vi "readUDP.vi"(8 "error in (no error)":errorcluster, 11 "Mockbus in":refnum<class "Mockbus.lvclass">) -> (0 "error out":errorcluster, 1 "CommandAvailable":bool, 2 "UDP Command":T1, 3 "Mockbus out":refnum<class "Mockbus.lvclass">)   [LabVIEW 2015, in "Mockbus.lvclass"]
uses:
  Mockbus.lvclass
  Typedefs/UDPCommand.ctl
  Mockbus.lvclass/Mockbus.ctl
  Typedefs/RTTypeDefs.lvlib
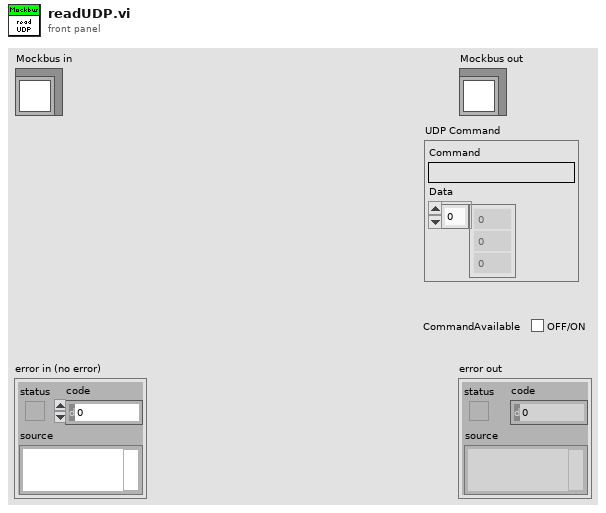
[diagram p1: front panel]
types:
  T1 = typedef "RTTypeDefs.lvlib/UDPCommand.ctl" = cluster{"Command":string, "Data":u8[]}
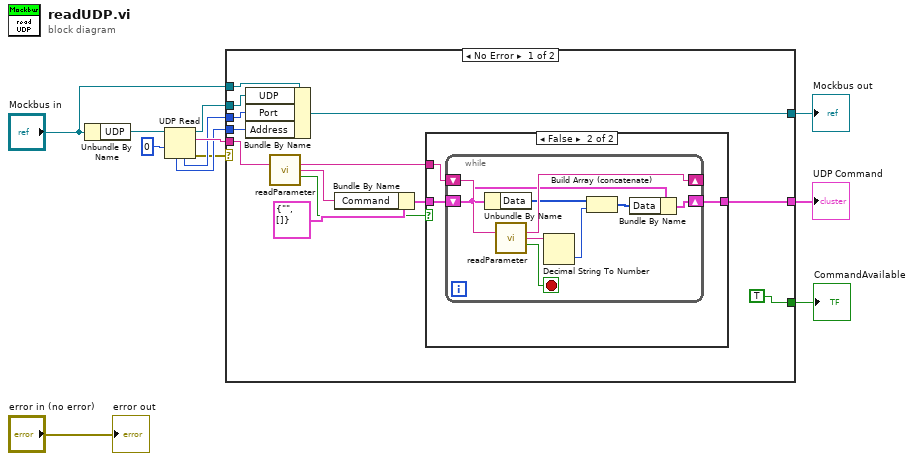
[diagram p0: block diagram]
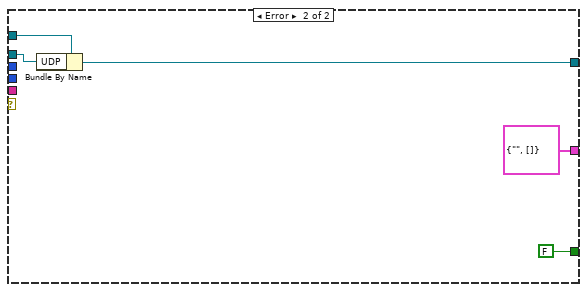
[diagram p3: hidden frame]
diagram:
  n1 = Unbundle By Name("Mockbus in") -> ("UDP"=w12:refnum<k16>)
  n2 = UDP Read(connection ID=w12, timeout ms (25000)=0) -> (data out=w11:string, error out=w3:errorcluster, 3:w9:refnum<k16>, 4:w7:u16, 6:w6:u32)  [unwired: 2 in]
  n3 = case shown="No Error" w3 {
    tunnel: w11 -> [w25 _]
    tunnel: "Mockbus in" -> [w19 w43]
    tunnel: w9 -> [w18 w42]
    tunnel: w7 -> [w17 _]
    tunnel: w6 -> [w16 _]
    tunnel: [w15 T1 {"Command"="", "Data"=[]} ("UDP Command")] -> w5
    tunnel: [w14 w41] -> w4
    tunnel: [TRUE FALSE] -> w1
    frame No Error {
      n4 = Bundle By Name(cluster=w19, "UDP"=w18, "Port"=w17, "Address"=w16) -> (w14:refnum<class "Mockbus.lvclass">)
      n5 = call "readParameter.vi"("Input"=w25) -> ("Output"=w24:string, "Parameter"=w22:string, "LastParameter?"=w20:bool)  [unwired: 10 in, 2 out]
      n6 = Bundle By Name(cluster=T1 {"Command"="", "Data"=[]} ("UDP Command"), "Command"=w22) -> (w21:T1)
      n7 = case shown="False" w20 {
        tunnel: w24 -> [_ w29]
        tunnel: w21 -> [w26 w28]
        tunnel: [w26 w27] -> w15
        frame True {
        }
        frame False {
          n8 = while {
            shift-right: [w37] -> _
            shift-left: w29 -> [w38]
            shift-right: [w30] -> w27
            shift-left: w28 -> [w31]
            stop <- w36 stop-if-true
            n9 = Unbundle By Name(w31) -> ("Data"=w34:u8[])
            n10 = call "readParameter.vi"("Input"=w38) -> ("Output"=w37:string, "Parameter"=w35:string, "LastParameter?"=w36:bool)  [unwired: 10 in, 2 out]
            n11 = Decimal String To Number(string=w35) -> (number=w33:i32)  [unwired: 2 in, 1 out]
            n12 = Build Array (concatenate)(w34, w33) -> (w32:i32[])
            n13 = Bundle By Name(cluster=w31, "Data"=w32) -> (w30:T1)
          }
        }
      }
    }
    frame Error {
      n14 = Bundle By Name(cluster=w43, "UDP"=w42) -> (w41:refnum<class "Mockbus.lvclass">)
    }
  }
  "Mockbus out" <- w4
  "UDP Command" <- w5
  "CommandAvailable" <- w1
  "error out" <- "error in (no error)"
